vi "Access insert values.vi"(5 "是否创建唯一键":bool, 6 "Password":string, 7 "data":variant[](array[variant]), 8 "error in (no error)":errorcluster, 9 "columns外部输入":T1, 10 "database":string="database1.mdb", 11 "table":string) -> (0 "error out":errorcluster)   [LabVIEW 2016, in "Access Lib.lvlib"]
uses:
  Access Lib.lvlib
  <vilib>/addons/database/Auxilliary.llb/DB Tools Transaction.ctl
  <vilib>/addons/database/Auxilliary.llb/DB Tools Isolation Level.ctl
  <vilib>/addons/database/Auxilliary.llb/DB Tools Column Info.ctl
  <vilib>/addons/database/Auxilliary.llb/DB Tools DataTypes.ctl
  <vilib>/addons/database/Auxilliary.llb/DB Tools Parameter Info.ctl
  <vilib>/addons/database/Auxilliary.llb/DB Tools Parameter Dir.ctl
  <vilib>/addons/database/Connection.llb/DB Tools Open Connec (String).vi
  <vilib>/addons/database/Connection.llb/Conn Transaction.vi
  <vilib>/addons/database/Connection.llb/Conn Execute.vi
  <vilib>/addons/database/Recordset.llb/Rec Destroy - Connection.vi
  <vilib>/addons/database/Command.llb/Cmd Set Parameter Value (C).vi
  <vilib>/addons/database/Command.llb/Cmd Execute.vi
  <vilib>/addons/database/Recordset.llb/Rec Destroy - Command.vi
  <vilib>/addons/database/Command.llb/Cmd Delete.vi
  <vilib>/addons/database/NI_Database_API.lvlib
  <vilib>/Utility/VariantDataType/VariantType.lvlib
panel:
  out "SN":string
  out "布尔":bool
  out "曲线截距":sgl
  out "曲线斜率":sgl
  out "二次多项式系数":sgl
  out "X":sgl
  out "检测值":sgl
  out "测试模式":enum16{"水样测试", "零点核查", "跨度核查"}(ring)
  out "当前数据时间":timestamp
  out "当前测量模式":string
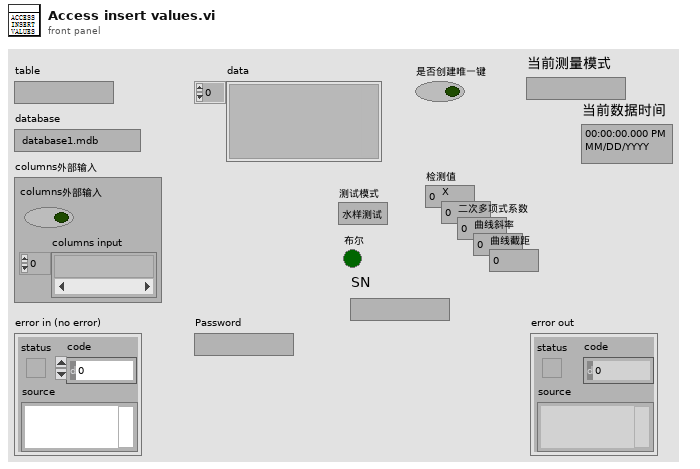
[diagram p1: front panel]
types:
  T1 = cluster{"columns外部输入":bool, "columns input":string[]}
  T2 = typedef "NI_Database_API.lvlib/DB Tools Isolation Level.ctl" = enum16{"chaos", "read uncommitted", "read committed", "repeatable read", "serializable"}
  T3 = typedef "NI_Database_API.lvlib/DB Tools Transaction.ctl" = enum16{"begin", "commit", "rollback"}
  T4 = typedef "NI_Database_API.lvlib/DB Tools Column Info.ctl" = cluster{"column name":string, "data type":T5, "size":i32, "allow null?":bool}
  T5 = typedef "NI_Database_API.lvlib/DB Tools DataTypes.ctl" = enum16{"String", "Long (I32)", "Single (SGL)", "Double (DBL)", "Date/Time", "Binary"}
  T6 = typedef "VariantType.lvlib/Type.ctl" = enum8{"Invalid Type", "Void", "I8", "I16", "I32", "I64", "U8", "U16", "U32", "U64", "Single Float", "Double Float", "Extended Float", "Single Complex", "Double Complex", "Extended Complex", "Enum U8", "Enum U16", "Enum U32", "Enum U64", "Single Float With Unit", "Double Float With Unit", "Extended Float With Unit", "Single Complex with Unit", "Double Complex with Unit", "Extended Complex with Unit", "Boolean", "String", "Path", "Picture", "Tag", "Array", "Cluster", "Variant", "LV Variant", "Waveform", "Timestamp", "Digital Waveform", "Digital Data", "ExpressData", "Refnum", "External Data", "VI", "Poly VI", "LabVIEW Class Instance", "Fixed Point"}
  T7 = typedef "NI_Database_API.lvlib/Conn ObjectReference.ctl" = refnum<k1>
  T8 = typedef "NI_Database_API.lvlib/DB Tools Parameter Info.ctl" = cluster{"parameter name":string, "type":T5, "direction":T9, "value":variant}
  T9 = typedef "NI_Database_API.lvlib/DB Tools Parameter Dir.ctl" = enum32{"Input", "Output", "Input/Output", "Return Value"}
  T10 = typedef "NI_Database_API.lvlib/Rec ObjectReference.ctl" = refnum<k1>
  T11 = typedef "LVDateTimeRec.ctl" = cluster{"秒数的小数部分":dbl, "秒":i32, "分":i32, "时":i32, "日":i32, "月":i32, "年":i32, "天数（周）":i32, "天数（年）":i32, "DST":i32}
  T12 = typedef "NI_Database_API.lvlib/Cmd ObjectReference.ctl" = refnum<k1>
  T13 = typedef "NI_Database_API.lvlib/Cmd-Rec Object Reference.ctl" = refnum<k1>
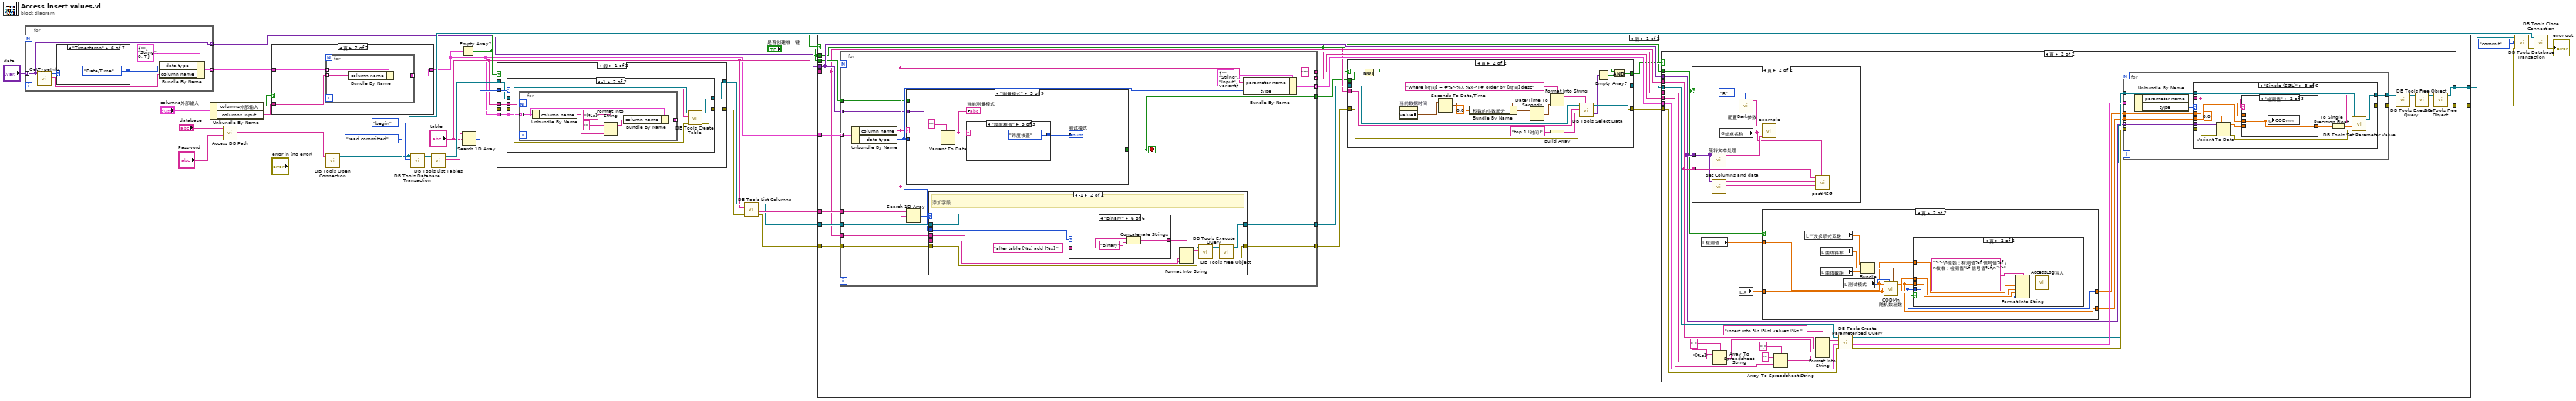
[diagram p0: block diagram]
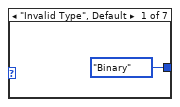
[diagram p3: hidden frame]
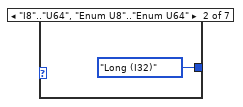
[diagram p4: hidden frame]
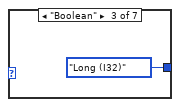
[diagram p5: hidden frame]
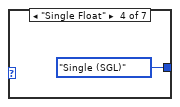
[diagram p6: hidden frame]
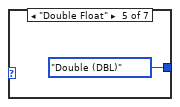
[diagram p7: hidden frame]
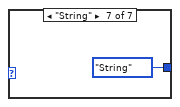
[diagram p8: hidden frame]
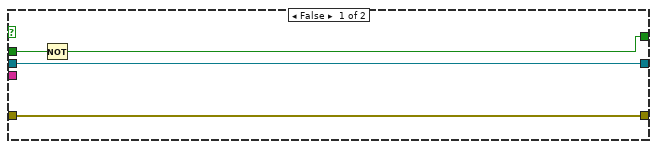
[diagram p11: hidden frame]
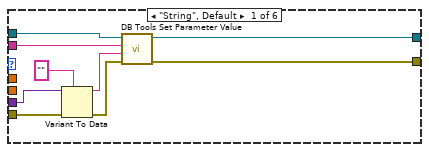
[diagram p16: hidden frame]
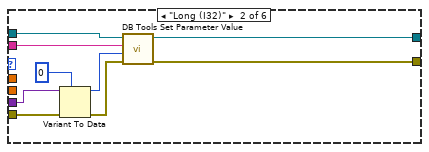
[diagram p17: hidden frame]
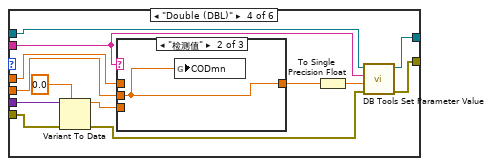
[diagram p20: hidden frame]
diagram:
  n1 = for {
    tunnel: [w35] -> w12 mode=indexing
    tunnel: [w37] -> w9 mode=indexing
    tunnel: "data" -> [w35] mode=indexing
    n2 = call <vilib>:"GetTypeInfo.vi"("Variant"=w35) -> ("Name"=w36:string, "Type Enum"=w39:T6)  [unwired: 6 in, 3 out]
    n3 = case shown="\"Timestamp\"" w39 {
      tunnel: [DB_Tools_DataTypes."Binary" ("data type") DB_Tools_DataTypes."Long (I32)" ("data type") DB_Tools_DataTypes."Long (I32)" ("data type") DB_Tools_DataTypes."Single (SGL)" ("data type") DB_Tools_DataTypes."Double (DBL)" ("data type") DB_Tools_DataTypes."Date/Time" ("data type") DB_Tools_DataTypes."String" ("data type")] -> w38
      frame "Invalid Type", Default {
      }
      frame "I8".."U64", "Enum U8".."Enum U64" {
      }
      frame "Boolean" {
      }
      frame "Single Float" {
      }
      frame "Double Float" {
      }
      frame "Timestamp" {
      }
      frame "String" {
      }
    }
    n4 = Bundle By Name(cluster=T4 {"column name"="", "data type"=enum."String", "size"=0, "allow null?"=TRUE} ("column information"), "data type"=w38, "column name"=w36) -> (w37:T4)
  }
  n5 = Unbundle By Name("columns外部输入") -> ("columns外部输入"=w7:bool, "columns input"=w8:string[])
  n6 = call "Access DB Path.vi"("Password"="Password", "database"="database") -> ("Connection information"=w5:string)  [unwired: 8 in, 1 out]
  n7 = case shown="真" w7 {
    tunnel: w9 -> [w48 w51]
    tunnel: [w48 w50] -> w6
    tunnel: w8 -> [_ w49]
    frame False {
    }
    frame True {
      n8 = for {
        tunnel: w51 -> [w54] mode=indexing
        tunnel: [w53] -> w50 mode=indexing
        tunnel: w49 -> [w52] mode=indexing
        n9 = Bundle By Name(cluster=w54, "column name"=w52) -> (w53:T4)
      }
    }
  }
  n10 = call-poly <vilib>:"DB Tools Open Connection.vi"("error in (no error)"="error in (no error)", "connection information"=w5) -> ("error out"=w19:errorcluster, "connection reference"=w16:T7)  [unwired: 6 in]
  n11 = call-poly <vilib>:"DB Tools Database Transaction.vi"("error in (no error)"=w19, "isolation level (chaos)"=DB_Tools_Isolation_Level."read committed", "operation (begin)"=DB_Tools_Transaction."begin", "connection reference"=w16) -> ("error out"=w18:errorcluster, "connection reference out"=w20:T7)  [unwired: 2 in]
  n12 = call <vilib>:"DB Tools List Tables.vi"("error in (no error)"=w18, "connection reference"=w20) -> ("error out"=w27:errorcluster, "tables"=w29:string[], "connection reference out"=w17:T7)  [unwired: 3 in]
  n13 = Empty Array?(array=w6) -> (empty?=w14:bool)
  n14 = Search 1D Array(1D array=w29, element="table") -> (index of element=w28:i32)  [unwired: 1 in]
  n15 = case shown="假" w14 {
    tunnel: w28 -> [w61 _]
    tunnel: w27 -> [w60 w77]
    tunnel: [w59 w78] -> w25
    tunnel: [w58 w77] -> w24
    tunnel: w17 -> [w57 w78]
    tunnel: "table" -> [w56 _]
    tunnel: w6 -> [w55 _]
    frame False {
      n16 = case shown="-1" w61 {
        tunnel: w57 -> [w63 w70]
        tunnel: w60 -> [w62 w69]
        tunnel: w56 -> [_ w68]
        tunnel: w55 -> [_ w65]
        tunnel: [w63 w67] -> w59
        tunnel: [w62 w66] -> w58
        frame 0, Default {
        }
        frame -1 {
          n17 = for {
            tunnel: w65 -> [w72] mode=indexing
            tunnel: [w71] -> w64 mode=indexing
            n18 = Unbundle By Name(w72) -> ("column name"=w76:string)
            n19 = Format Into String(format string="[%s]" ("格式字符串"), initial string="" ("初始字符串"), w76) -> (resulting string=w73:string)  [unwired: 1 in, 1 out]
            n20 = Bundle By Name(cluster=w72, "column name"=w73) -> (w71:T4)
          }
          n21 = call <vilib>:"DB Tools Create Table.vi"("error in (no error)"=w69, "column information"=w64, "table"=w68, "connection reference"=w70) -> ("error out"=w66:errorcluster, "connection reference out"=w67:T7)  [unwired: 4 in]
        }
      }
    }
    frame True {
    }
  }
  n22 = call <vilib>:"DB Tools List Columns.vi"("error in (no error)"=w24, "table"="table", "connection reference"=w25) -> ("error out"=w3:errorcluster, "columns"=w26:string[], "connection reference out"=w4:T7)  [unwired: 1 in, 1 out]
  n23 = case shown="假" w14 {
    tunnel: w26 -> [w97 _]
    tunnel: w3 -> [w96 w345]
    tunnel: [w92 w346] -> w22
    tunnel: [w91 w345] -> w21
    tunnel: w12 -> [w88 _]
    tunnel: w4 -> [w90 w346]
    tunnel: "table" -> [w82 _]
    tunnel: w6 -> [w89 _]
    tunnel: "是否创建唯一键" -> [w87 _]
    tunnel: "是否创建唯一键" -> [w79 _]
    frame False {
      n24 = for {
        tunnel: w90 -> [w275]
        tunnel: w97 -> [w277]
        tunnel: w96 -> [w274]
        tunnel: [w273] -> w84
        tunnel: w82 -> [w272]
        tunnel: w89 -> [w271] mode=indexing
        tunnel: [w269] -> w95 mode=indexing
        tunnel: [w265] -> w94 mode=indexing
        tunnel: ["?"] -> w93 mode=indexing
        tunnel: [w267] -> w86
        tunnel: w88 -> [w264] mode=indexing
        tunnel: [w263] -> w81
        tunnel: w87 -> [w262]
        stop <- w263 stop-if-true
        n25 = Unbundle By Name(w271) -> ("column name"=w265:string, "data type"=w266:T5)
        n26 = case shown="\"测量模式\"" w265 {
          tunnel: w266 -> [_ w281 _ _ _ _ _ _ _]
          tunnel: w264 -> [_ w280 w290 w296 w299 w302 w305 w308 w311]
          tunnel: [_ w279 _ _ _ _ _ _ _] -> w263
          tunnel: w262 -> [_ w278 _ _ _ _ _ _ _]
          frame "假", Default {
          }
          frame "时间" {
            n27 = case shown="\"Date/Time\"" w281 {
              tunnel: w280 -> [_ w286]
              tunnel: [_ w282] -> w279
              tunnel: w278 -> [_ _]
              frame "String", Default {
              }
              frame "Date/Time" {
                n28 = Variant To Data(type=timestamp(0 s since 1904-01-01) ("时间标识"), Variant=w286) -> (data=w284:timestamp)  [unwired: 1 in, 1 out]
                "当前数据时间" <- w284
                n29 = Equal?(x=w284, y=timestamp(0 s since 1904-01-01) ("时间标识")) -> (x = y?=w282:bool)
              }
            }
          }
          frame "测量模式" {
            n30 = Variant To Data(type="", Variant=w290) -> (data=w288:string)  [unwired: 1 in, 1 out]
            "当前测量模式" <- w288
            n31 = case shown="\"跨度核查\"" w288 {
              tunnel: [enum16{"水样测试", "零点核查", "跨度核查"}."水样测试" ("测试模式") enum16{"水样测试", "零点核查", "跨度核查"}."零点核查" ("测试模式") enum16{"水样测试", "零点核查", "跨度核查"}."跨度核查" ("测试模式")] -> w287
              frame "水样测试", Default {
              }
              frame "零点核查" {
              }
              frame "跨度核查" {
              }
            }
            "测试模式" <- w287
          }
          frame "检测值" {
            n32 = Variant To Data(type=sgl 0.0, Variant=w296) -> (data=→"检测值":sgl)  [unwired: 1 in, 1 out]
            "布尔" <- TRUE ("布尔")
          }
          frame "X0" {
            n33 = Variant To Data(type=sgl 0.0, Variant=w299) -> (data=→"X":sgl)  [unwired: 1 in, 1 out]
          }
          frame "二次多项式系数" {
            n34 = Variant To Data(type=sgl 0.0, Variant=w302) -> (data=→"二次多项式系数":sgl)  [unwired: 1 in, 1 out]
          }
          frame "曲线斜率" {
            n35 = Variant To Data(type=sgl 0.0, Variant=w305) -> (data=→"曲线斜率":sgl)  [unwired: 1 in, 1 out]
          }
          frame "曲线截距" {
            n36 = Variant To Data(type=sgl 0.0, Variant=w308) -> (data=→"曲线截距":sgl)  [unwired: 1 in, 1 out]
          }
          frame "SN" {
            n37 = Variant To Data(type="", Variant=w311) -> (data=→"SN":string)  [unwired: 1 in, 1 out]
          }
        }
        n38 = Search 1D Array(1D array=w277, element=w265) -> (index of element=w276:i32)  [unwired: 1 in]
        n39 = case shown="-1" w276 {
          tunnel: [w314 w323] -> w273
          tunnel: w275 -> [w313 w322]
          tunnel: w265 -> [_ w321]
          tunnel: w274 -> [w314 w320]
          tunnel: w272 -> [_ w319]
          tunnel: w266 -> [_ w317]
          tunnel: [w313 w315] -> w267
          frame 0, Default {
          }
          frame -1 {
            # "添加字段"
            n40 = case shown="\"Binary\"" w317 {
              tunnel: "alter table [%s] add [%s] " -> [w329 w332 w335 w338 w341 w344]
              tunnel: [w328 w331 w334 w337 w340 w343] -> w316
              frame "String", Default {
                n41 = Concatenate Strings(w329, "String" ("字符串")) -> (w328:string)
              }
              frame "Long (I32)" {
                n42 = Concatenate Strings(w332, "Long" ("字符串")) -> (w331:string)
              }
              frame "Single (SGL)" {
                n43 = Concatenate Strings(w335, "Single" ("字符串")) -> (w334:string)
              }
              frame "Double (DBL)" {
                n44 = Concatenate Strings(w338, "Double" ("字符串")) -> (w337:string)
              }
              frame "Date/Time" {
                n45 = Concatenate Strings(w341, "TimeStamp" ("字符串")) -> (w340:string)
              }
              frame "Binary" {
                n46 = Concatenate Strings(w344, "Binary" ("字符串")) -> (w343:string)
              }
            }
            n47 = Format Into String(format string=w316, w319, w321) -> (resulting string=w324:string)  [unwired: 2 in, 1 out]
            n48 = call-poly <vilib>:"DB Tools Execute Query.vi"("error in (no error)"=w320, "SQL query"=w324, "connection reference"=w322) -> ("error out"=w325:errorcluster, "recordset reference"=w326:T10)  [unwired: 5 in]
            n49 = call-poly <vilib>:"DB Tools Free Object.vi"("error in (no error)"=w325, "recordset reference"=w326) -> ("error out"=w323:errorcluster, "connection reference"=w315:T7)  [unwired: 8 in]
          }
        }
        n50 = Bundle By Name(cluster=T8 {"parameter name"="", "type"=enum."String", "direction"=enum."Input", "value"=variant} ("parameter information"), "parameter name"=w265, "type"=w266) -> (w269:T8)
      }
      n51 = case shown="真" w79 {
        tunnel: w86 -> [w101 w118]
        tunnel: [w101 w117] -> w85
        tunnel: w84 -> [w100 w116]
        tunnel: [w100 w115] -> w83
        tunnel: w82 -> [_ w114]
        tunnel: w81 -> [w99 w103]
        tunnel: [w98 w105] -> w80
        frame False {
          n52 = Not(x=w99) -> (.not. x?=w98:bool)
        }
        frame True {
          n53 = Not(x=w103) -> (.not. x?=w102:bool)
          n54 = property on="当前数据时间" class="AbsTime (严格)"() -> ("Value"=w111:timestamp)  [unwired: 2 in, 2 out]
          n55 = Seconds To Date/Time(time stamp (now)=w111) -> (date time rec=w110:T11)  [unwired: 1 in]
          n56 = Bundle By Name(cluster=w110, "秒数的小数部分"=0.0) -> (w107:T11)
          n57 = Date/Time To Seconds(2:w107) -> (0:w108:timestamp)  [unwired: 1 in]
          n58 = Format Into String(format string="where [时间] = #%<%X %x>T# order by [时间] desc" ("condition"), w108) -> (resulting string=w113:string)  [unwired: 2 in, 1 out]
          n59 = Build Array("top 1 [时间]") -> (w120:string[])
          n60 = call <vilib>:"DB Tools Select Data.vi"("condition"=w113, "error in (no error)"=w116, "columns"=w120, "table"=w114, "connection reference"=w118) -> ("error out"=w115:errorcluster, "data"=w106:variant[][], "connection reference out"=w117:T7)  [unwired: 1 in]
          n61 = Empty Array?(array=w106) -> (empty?=w104:bool)
          n62 = And(x=w102, y=w104) -> (x .and. y?=w105:bool)
        }
      }
      n63 = case shown="真" w80 {
        tunnel: w95 -> [_ w153]
        tunnel: w94 -> [_ w147]
        tunnel: w93 -> [_ w145]
        tunnel: [w122 w135] -> w92
        tunnel: [w121 w134] -> w91
        tunnel: w85 -> [w122 w132]
        tunnel: w83 -> [w121 w130]
        tunnel: w82 -> [_ w125]
        tunnel: w88 -> [_ w124]
        tunnel: w79 -> [_ w123]
        frame False {
        }
        frame True {
          n64 = case shown="真" w123 {
            tunnel: w125 -> [_ w159]
            tunnel: w124 -> [_ w158]
            frame False {
            }
            frame True {
              n65 = call "簇转文本处理.vi"("data"=w158) -> ("output"=w157:string)  [unwired: 10 in]
              n66 = call "get Columns and data.vi"("数组"=w158) -> ("data"=w160:string[], "columns"=w161:string[])  [unwired: 9 in]
              n67 = global read "系统全局.vi" "站点名称"() -> (w156:string)
              n68 = call "配置Bark参数.vi"("FUN"=enum16{"W", "R"}."R") -> ("URLs 2"=w154:string[])  [unwired: 10 in]
              n69 = call "example.vi"("Message"=w157, "Title"=w156, "Group"=w156, "urls"=w154) -> ()  [unwired: 8 in]
              n70 = call "postMSG.vi"("station"=w156, "data"=w160, "columns"=w161, "table"=w159) -> ()  [unwired: 7 in, 1 out]
            }
          }
          n71 = local read "检测值"() -> (w129:sgl)
          n72 = Array To Spreadsheet String(delimiter (Tab)="," ("分隔符(Tab)"), array=w147, 3:"[%s]" ("格式字符串")) -> (spreadsheet string=w146:string)
          n73 = local read "X"() -> (w128:sgl)
          n74 = case shown="真" w123 {
            tunnel: w129 -> [w163 w167]
            tunnel: w128 -> [w162 w166]
            tunnel: [w163 w165] -> w127
            tunnel: [w162 w164] -> w126
            frame False {
            }
            frame True {
              n75 = local read "二次多项式系数"() -> (w173:sgl)
              n76 = local read "曲线斜率"() -> (w172:sgl)
              n77 = local read "曲线截距"() -> (w171:sgl)
              n78 = local read "测试模式"() -> (w169:enum16{"水样测试", "零点核查", "跨度核查"})
              n79 = Bundle("二次多项式系数"=w173, "曲线斜率"=w172, "曲线截距"=w171) -> (w170:cluster{"二次多项式系数":sgl, "曲线斜率":sgl, "曲线截距":sgl})  [unwired: 1 in]
              n80 = call "CODMn 随机数出数.vi"("公式"=w170, "测试模式"=w169, "信号值原始值"=w166, "原始值"=w167) -> ("随机数？"=w168:bool, "信号值"=w164:u16, "取值输出"=w165:dbl)  [unwired: 3 in]
              n81 = case shown="真" w168 {
                tunnel: w167 -> [_ w177]
                tunnel: w166 -> [_ w176]
                tunnel: w165 -> [_ w175]
                tunnel: w164 -> [_ w174]
                frame False {
                }
                frame True {
                  n82 = Format Into String(format string="<<\n原始：检测值%f 信号值%f \n校准：检测值%f 信号值%f\n>>" ("格式字符串"), w177, w176, w175, w174) -> (resulting string=w178:string)  [unwired: 2 in, 1 out]
                  n83 = call "AccessLog写入.vi"("Log"=w178) -> ()  [unwired: 11 in]
                }
              }
            }
          }
          n84 = Array To Spreadsheet String(delimiter (Tab)="," ("分隔符(Tab)"), array=w145, 3:"" ("格式字符串")) -> (spreadsheet string=w144:string)
          n85 = Format Into String(format string="insert into %s (%s) values (%s)" ("格式字符串"), w125, w146, w144) -> (resulting string=w143:string)  [unwired: 2 in, 1 out]
          n86 = call <vilib>:"DB Tools Create Parameterized Query.vi"("error in (no error)"=w130, "parameters"=w153, "SQL query"=w143, "connection reference"=w132) -> ("error out"=w142:errorcluster, "parameters out"=w141:T8[], "command reference"=w133:T12)  [unwired: 3 in]
          n87 = for {
            tunnel: w133 -> [w186]
            tunnel: w142 -> [w184]
            tunnel: w141 -> [w189] mode=indexing
            tunnel: w124 -> [w187] mode=indexing
            tunnel: [w183] -> w131
            tunnel: [w182] -> w140
            tunnel: w127 -> [w181]
            tunnel: w126 -> [w180]
            n88 = Unbundle By Name(w189) -> ("parameter name"=w185:string, "type"=w188:T5)
            n89 = case shown="\"Single (SGL)\"" w188 {
              tunnel: w187 -> [w193 w201 w214 w230 w249 w253]
              tunnel: w186 -> [w196 w205 w217 w234 w247 w261]
              tunnel: w185 -> [w195 w204 w213 w229 w242 w260]
              tunnel: w184 -> [w190 w199 w215 w231 w245 w252]
              tunnel: [w192 w203 w218 w233 w244 w259] -> w183
              tunnel: [w191 w202 w216 w232 w243 w258] -> w182
              tunnel: w181 -> [_ _ w211 w228 _ _]
              tunnel: w180 -> [_ _ w212 w227 _ _]
              frame "String", Default {
                n90 = Variant To Data(error in=w190, type="", Variant=w193) -> (data=w194:string, error out=w198:errorcluster)
                n91 = call-poly <vilib>:"DB Tools Set Parameter Value.vi"("error in (no error)"=w198, "value"=w194, "parameter index"=w195, "command reference"=w196) -> ("error out"=w191:errorcluster, "command reference out"=w192:T12)  [unwired: 4 in]
              }
              frame "Long (I32)" {
                n92 = Variant To Data(error in=w199, type=0, Variant=w201) -> (data=w206:i32, error out=w207:errorcluster)
                n93 = call-poly <vilib>:"DB Tools Set Parameter Value.vi"("error in (no error)"=w207, "value"=w206, "parameter index"=w204, "command reference"=w205) -> ("error out"=w202:errorcluster, "command reference out"=w203:T12)  [unwired: 4 in]
              }
              frame "Single (SGL)" {
                n94 = Variant To Data(error in=w215, type=sgl 0.0, Variant=w214) -> (data=w210:sgl, error out=w220:errorcluster)
                n95 = case shown="\"检测值\"" w213 {
                  tunnel: w211 -> [_ w222 _]
                  tunnel: w210 -> [w221 _ _]
                  tunnel: [w221 w222 w223] -> w209
                  tunnel: w212 -> [_ _ w223]
                  frame Default {
                  }
                  frame "检测值" {
                    n96 = global write "系统全局.vi" "CODmn"(w222) -> ()
                  }
                  frame "X0", "测量信号值" {
                  }
                }
                n97 = To Single Precision Float(number=w209) -> (single precision float=w208:sgl)
                n98 = call-poly <vilib>:"DB Tools Set Parameter Value.vi"("error in (no error)"=w220, "value"=w208, "parameter index"=w213, "command reference"=w217) -> ("error out"=w216:errorcluster, "command reference out"=w218:T12)  [unwired: 4 in]
              }
              frame "Double (DBL)" {
                n99 = Variant To Data(error in=w231, type=0.0, Variant=w230) -> (data=w226:dbl, error out=w236:errorcluster)
                n100 = case shown="\"检测值\"" w229 {
                  tunnel: w228 -> [_ w238 _]
                  tunnel: w226 -> [w237 _ _]
                  tunnel: [w237 w238 w239] -> w225
                  tunnel: w227 -> [_ _ w239]
                  frame Default {
                  }
                  frame "检测值" {
                    n101 = global write "系统全局.vi" "CODmn"(w238) -> ()
                  }
                  frame "X0", "测量信号值" {
                  }
                }
                n102 = To Single Precision Float(number=w225) -> (single precision float=w224:sgl)
                n103 = call-poly <vilib>:"DB Tools Set Parameter Value.vi"("error in (no error)"=w236, "value"=w224, "parameter index"=w229, "command reference"=w234) -> ("error out"=w232:errorcluster, "command reference out"=w233:T12)  [unwired: 4 in]
              }
              frame "Date/Time" {
                n104 = Variant To Data(error in=w245, type=timestamp(0 s since 1904-01-01) ("时间标识"), Variant=w249) -> (data=w241:timestamp, error out=w246:errorcluster)
                n105 = Format Date/Time String(seconds (now)=w241) -> (date/time string=w240:string)  [unwired: 2 in]
                n106 = call-poly <vilib>:"DB Tools Set Parameter Value.vi"("error in (no error)"=w246, "value"=w240, "parameter index"=w242, "command reference"=w247) -> ("error out"=w243:errorcluster, "command reference out"=w244:T12)  [unwired: 4 in]
              }
              frame "Binary" {
                n107 = Variant To Flattened String(Variant=w253) -> (data string=w254:string)  [unwired: 1 out]
                n108 = String To Byte Array(string=w254) -> (unsigned byte array=w257:u8[])
                n109 = Set Variant Attribute(Variant=w257, name="flat", value=TRUE, error in=w252) -> (Variant out=w250:variant, error out=w251:errorcluster)  [unwired: 1 out]
                n110 = call-poly <vilib>:"DB Tools Set Parameter Value.vi"("error in (no error)"=w251, "value"=w250, "parameter index"=w260, "command reference"=w261) -> ("error out"=w258:errorcluster, "command reference out"=w259:T12)  [unwired: 4 in]
              }
            }
          }
          n111 = call-poly <vilib>:"DB Tools Execute Query.vi"("error in (no error)"=w140, "command reference"=w131) -> ("error out"=w138:errorcluster, "command-recordset reference"=w139:T13)  [unwired: 6 in]
          n112 = call-poly <vilib>:"DB Tools Free Object.vi"("error in (no error)"=w138, "command-recordset reference"=w139) -> ("error out"=w136:errorcluster, "command reference"=w137:T12)  [unwired: 8 in]
          n113 = call-poly <vilib>:"DB Tools Free Object.vi"("error in (no error)"=w136, "command reference"=w137) -> ("error out"=w134:errorcluster, "connection reference"=w135:T7)  [unwired: 8 in]
        }
      }
    }
    frame True {
    }
  }
  n114 = call-poly <vilib>:"DB Tools Database Transaction.vi"("error in (no error)"=w21, "operation (begin)"=DB_Tools_Transaction."commit", "connection reference"=w22) -> ("error out"=w23:errorcluster)  [unwired: 3 in, 1 out]
  n115 = call <vilib>:"DB Tools Close Connection.vi"("error in (no error)"=w23, "connection reference"=w16) -> ("error out"=→"error out":errorcluster)  [unwired: 5 in]
